vi "Hit Detection.vi"(6 "Button":u16, 8 "error in (no error)":errorcluster, 9 "Alt button?":bool, 10 "Coords":T1, 11 "SceneGraphDisp Refnum":refnum<vi>) -> (0 "error out":errorcluster, 1 "Surface hit?":bool, 3 "PickPoint":T2)   [LabVIEW 2023]
doc: "Detect a hit on the surface."
uses:
  <vilib>/Utility/miscctls.llb/LV3DPointTypeDef.ctl
  <vilib>/Utility/miscctls.llb/LVPoint32TypeDef.ctl
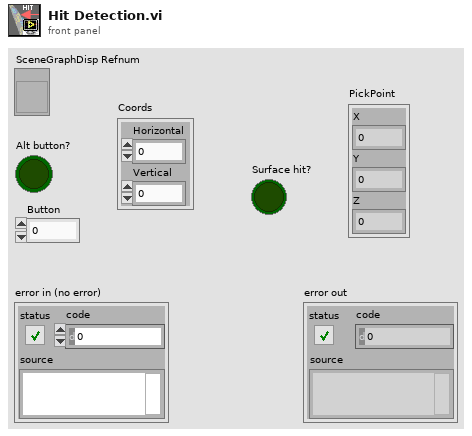
[diagram p1: front panel]
types:
  T1 = typedef "LVPoint32TypeDef.ctl" = cluster{"Horizontal":i32, "Vertical":i32}
  T2 = typedef "LV3DPointTypeDef.ctl" = cluster{"X":sgl, "Y":sgl, "Z":sgl}
  T3 = typedef "LVPositionTypeDef.ctl" = cluster{"Left":i32, "Top":i32}
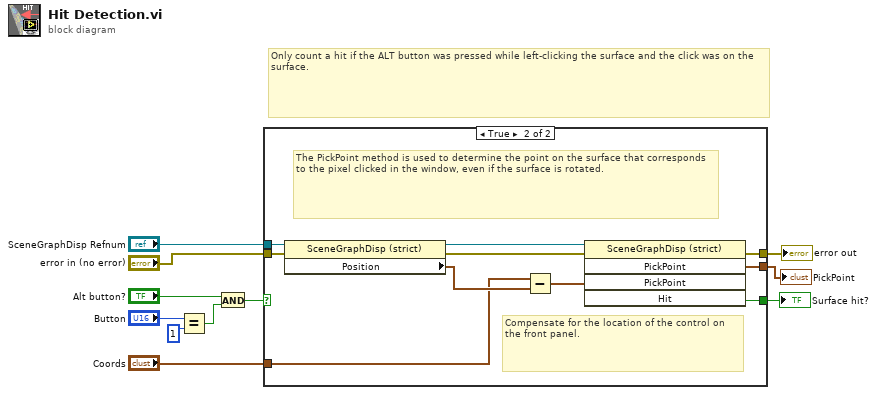
[diagram p0: block diagram]
diagram:
  # "Only count a hit if the ALT button was pressed while left-clicking the surface and the click was on the surface."
  n1 = Equal?(x="Button", y=u16 1) -> (x = y?=w9:bool)
  n2 = And(x="Alt button?", y=w9) -> (x .and. y?=w5:bool)
  n3 = case shown="True" w5 {
    selector: w5 -> [w13 _]
    tunnel: [_ w23] -> w11
    tunnel: [w13 w22] -> w10
    tunnel: "SceneGraphDisp Refnum" -> [_ w20]
    tunnel: "error in (no error)" -> [w12 w16]
    tunnel: [w12 w15] -> w2
    tunnel: "Coords" -> [_ w14]
    frame False {
    }
    frame True {
      # "The PickPoint method is used to determine the point on the surface that corresponds to the pixel clicked in the window, even if the surface is rotated."
      # "Compensate for the location of the control on the front panel."
      n4 = property on="Property Node" class="SceneGraphDisp (strict)"(reference=w20, error in=w16) -> (reference out=w19:refnum<vi>, error out=w18:errorcluster, "Position"=w21:T3)
      n5 = Subtract(x=w14, y=w21) -> (x-y=w17:T1)
      n6 = invoke on="Invoke Node" class="SceneGraphDisp (strict)" method="PickPoint"(reference=w19, error in=w18, "PickPoint"=w17) -> (error out=w15:errorcluster, "PickPoint"=w23:T2, "Hit"=w22:bool)  [unwired: 2 in, 2 out]
    }
  }
  "PickPoint" <- w11
  "Surface hit?" <- w10
  "error out" <- w2
